vi "ritter init.vi"(6 "Ritter Gas Drum Meter Enable":bool, 8 "error in (no error)":errorcluster, 11 "VISA in":refnum<visa-resource-name>) -> (0 "error out":errorcluster, 3 "VISA out":refnum<visa-resource-name>)   [LabVIEW 2020]
doc: "This vi open the connection to the gasmeter with default serial settings."
uses:
  <vilib>/Instr/_visa.llb/VISA Configure Serial Port (Instr).vi
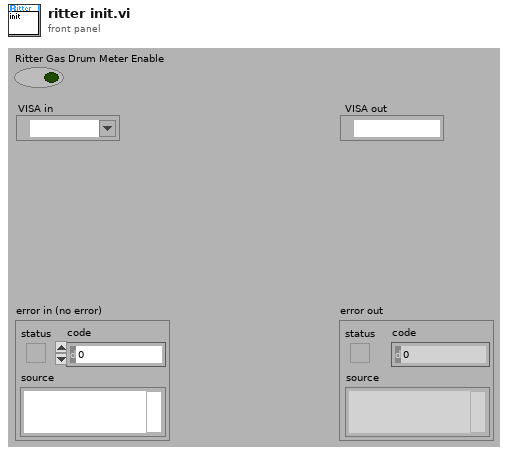
[diagram p1: front panel]
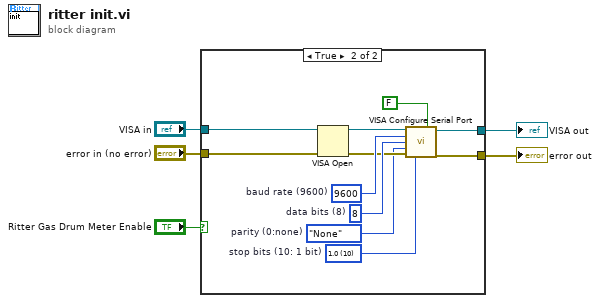
[diagram p0: block diagram]
diagram:
  n1 = case shown="True" "Ritter Gas Drum Meter Enable" {
    tunnel: "VISA in" -> [w6 w18]
    tunnel: [w6 w12] -> w4
    tunnel: [w7 w11] -> w3
    tunnel: "error in (no error)" -> [w7 w10]
    frame False {
    }
    frame True {
      w9 = enum16{"None", "Odd", "Even", "Mark", "Space"}."None"  # parity (0:none)
      w14 = u16 10 items=["1.0"=10, "1.5"=15, "2.0"=20]  # stop bits (10: 1 bit)
      w15 = u16 8  # data bits (8)
      w16 = u32 9600  # baud rate (9600)
      n2 = VISA Open(error in (no error)=w10, VISA resource name=w18) -> (VISA resource name=w17:refnum<visa-resource-name>, error out=w13:errorcluster)  [unwired: 3 in]
      n3 = call-poly "VISA Configure Serial Port"("VISA resource name"=w17, "Enable Termination\nChar (T)"=FALSE ("Enable Termination\nChar (T)"), "baud rate (9600)"=w16, "data bits (8)"=w15, "parity (0:none)"=w9, "error in (no error)"=w13, "stop bits (10: 1 bit)"=w14) -> ("VISA resource name out"=w12:refnum<visa-resource-name>, "error out"=w11:errorcluster)  [unwired: 7 in]
    }
  }
  "VISA out" <- w4
  "error out" <- w3
